vi "Actor Core.vi"(8 "error in":errorcluster, 11 "Nested in":refnum<class "ContadorB.lvclass">) -> (0 "error out":errorcluster, 3 "Actor out":refnum<class "Actor.lvclass">)   [LabVIEW 2019, in "ContadorB.lvlib" / "ContadorB.lvclass"]
doc: "(<B>Filename</B>: Actor Framework.lvlib:Actor.lvclass:Actor Core.vi)\n\nReceives messages to the actor, reacts to them, and initiates any error handling that may shut the actor down.\n\nDescendant classes may override this VI to append parallel tasks for the actor to complete while it handles messages. Overrides use the Call Parent Method node."
uses:
  ContadorB.lvclass
  C:/Program Files (x86)/National Instruments/LabVIEW 2019/vi.lib/ActorFramework/Actor/Actor.lvclass
  <vilib>/ActorFramework/Actor/Actor.lvclass
  startconteo/startconteo/startconteo.lvclass
  <vilib>/ActorFramework/Actor/Actor.lvclass/Actor.ctl
  <vilib>/ActorFramework/Message Enqueuer/Message Enqueuer.lvclass/Message Enqueuer.ctl
  ContadorB.lvclass/ContadorB.ctl
  startconteo/startconteo Messages/StartStop Msg/StartStop Msg.lvclass/StartStop Msg.ctl
  ContadorB Messages/contar Msg/contar Msg.lvclass/contar Msg.ctl
  startconteo/startconteo Messages/Maximo Msg/Maximo Msg.lvclass/Maximo Msg.ctl
  <vilib>/ActorFramework/Message Enqueuer/Init from Existing Queue.vi
  <vilib>/ActorFramework/Message Enqueuer/Enqueue.vi
  <vilib>/ActorFramework/Stop Msg/Stop Msg.lvclass
  C:/Program Files (x86)/National Instruments/LabVIEW 2019/vi.lib/ActorFramework/Message/Message.lvclass
  startconteo/startconteo Messages/StartStop Msg/StartStop Msg.lvclass
  ContadorB Messages/contar Msg/contar Msg.lvclass
  ContadorB Messages/stopcontar Msg/stopcontar Msg.lvclass
  startconteo/startconteo Messages/Maximo Msg/Maximo Msg.lvclass
  <vilib>/ActorFramework/Message Priority Queue/Priority Enqueue.vi
  <vilib>/ActorFramework/Message Enqueuer/Message Enqueuer.lvclass
panel:
  in  "Min":u8
  in  "Max":u8
  in  "Guardar":bool
  in  "Stop":bool
  in  "Start":bool
  out "Leds":bool[](array[boolean])
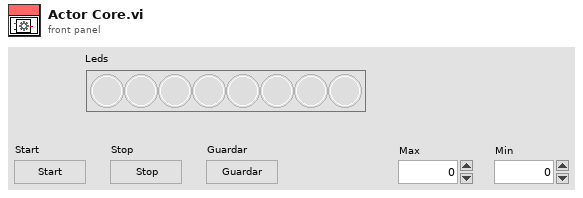
[diagram p1: front panel]
types:
  T1 = cluster{"Stop":refnum<user-event>, "Leds":refnum<user-event>}
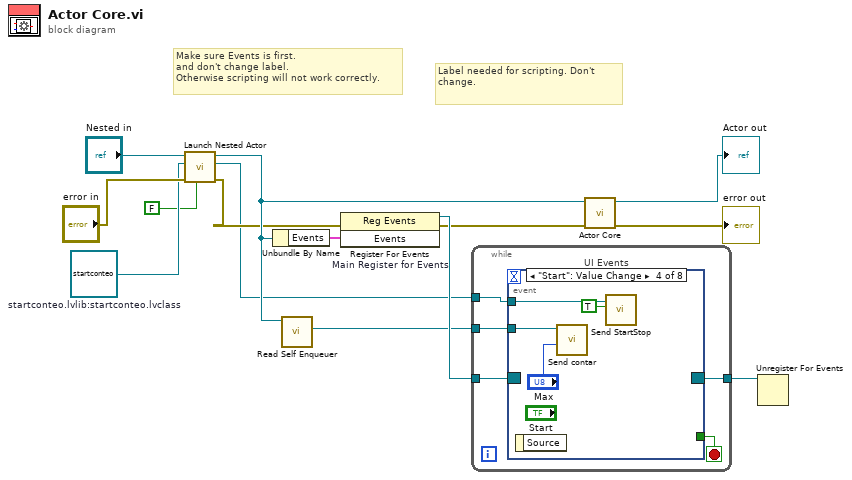
[diagram p0: block diagram]
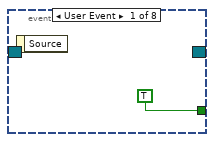
[diagram p2: hidden frame]
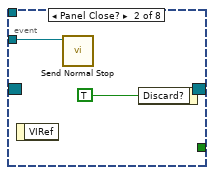
[diagram p3: hidden frame]
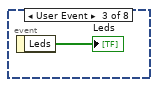
[diagram p4: hidden frame]
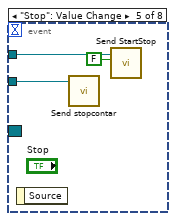
[diagram p5: hidden frame]
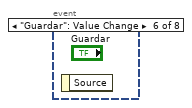
[diagram p6: hidden frame]
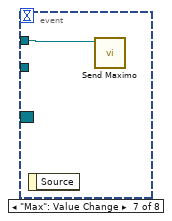
[diagram p7: hidden frame]
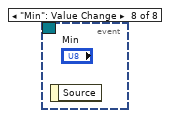
[diagram p8: hidden frame]
diagram:
  w3 = refnum<class "startconteo.lvclass"> refnum  # startconteo.lvlib:startconteo.lvclass
  # "Label needed for scripting. Don't change."
  # "Make sure Events is first.\nand don't change label.\nOtherwise scripting will not work correctly."
  n1 = call <vilib>:"Launch Nested Actor.vi"("Open Actor Core front panel? (F)"=FALSE ("Auto-stop? (T)"), "error in (no error)"="error in", "Nested Actor"=w3, "Caller Actor in"="Nested in") -> ("error out"=w4:errorcluster, "Nested Actor's Enqueuer"=w2:refnum<class "Message Enqueuer.lvclass">, "Caller Actor out"=w6:refnum<class "ContadorB.lvclass">)  [unwired: 5 in]
  n2 = Unbundle By Name(w6) -> ("Events"=w11:T1)
  n3 = call <vilib>:"Read Self Enqueuer.vi"("Actor"=w6) -> ("Self Enqueuer"=w9:refnum<class "Message Enqueuer.lvclass">)  [unwired: 10 in]
  n4 = register-events "Main Register for Events"(error in=w4, w11) -> (reference out=w12:refnum<event-registration>, error out=w8:errorcluster)  [unwired: 1 in]
  n5 = while {
    tunnel: w12 -> [w19]
    tunnel: [w17] -> w10
    tunnel: w9 -> [w16]
    tunnel: w2 -> [w15]
    stop <- w18 stop-if-true
    n6 = event "UI Events" shown="[3] \"Start\": Value Change" {
      selector: w19 -> [_ _ _ _ _ _ _ _]
      dyn-events: [_ _ _ _ _ _ _ _] -> w17
      timeout: _ -> [_ _ _ _ _ _ _ _]
      tunnel: [TRUE _ _ _ _ _ _ _] -> w18
      tunnel: w16 -> [_ w21 _ w27 w30 _ _ _]
      tunnel: w15 -> [_ _ _ w26 w29 _ w31 _]
      event User Event {
        n7 = event-data() -> ()  [unwired: 1 in, 1 out]
      }
      event Panel Close? {
        n8 = event-data() -> ()  [unwired: 1 in, 1 out]
        n9 = call <vilib>:"Send Normal Stop.vi"("Message Enqueuer"=w21) -> ()  [unwired: 10 in, 1 out]
        n10 = event-data("Discard?"=TRUE) -> ()  [unwired: 1 in, 1 out]
      }
      event User Event {
        n11 = event-data() -> ("Leds"=→"Leds":bool[])  [unwired: 1 in]
      }
      event "Start": Value Change {
        n12 = event-data() -> ()  [unwired: 1 in, 1 out]
        n13 = call "Send contar.vi"("Max"="Max", "Message Enqueuer"=w27) -> ()  [unwired: 8 in, 2 out]
        n14 = call "Send StartStop.vi"("StartStop"=TRUE, "Message Enqueuer"=w26) -> ()  [unwired: 8 in, 2 out]
      }
      event "Stop": Value Change {
        n15 = event-data() -> ()  [unwired: 1 in, 1 out]
        n16 = call "Send stopcontar.vi"("Message Enqueuer"=w30) -> ()  [unwired: 9 in, 2 out]
        n17 = call "Send StartStop.vi"("StartStop"=FALSE, "Message Enqueuer"=w29) -> ()  [unwired: 8 in, 2 out]
      }
      event "Guardar": Value Change {
        n18 = event-data() -> ()  [unwired: 1 in, 1 out]
      }
      event "Max": Value Change {
        n19 = event-data() -> ()  [unwired: 1 in, 1 out]
        n20 = call "Send Maximo.vi"("Message Enqueuer"=w31) -> ()  [unwired: 9 in, 2 out]
      }
      event "Min": Value Change {
        n21 = event-data() -> ()  [unwired: 1 in, 1 out]
      }
    }
  }
  n22 = call-parent "Actor Core.vi"("error in"=w8, "Actor in"=w6) -> ("error out"=→"error out":errorcluster, "Actor out"=→"Actor out":refnum<class "Actor.lvclass">)  [unwired: 8 in]
  n23 = Unregister For Events(event registration refnum=w10) -> ()  [unwired: 1 in, 1 out]
